vi "C867_Stop.vi"(8 "error in":errorcluster caption="entrée d'erreur") -> (0 "error out":errorcluster caption="sortie d'erreur")   [LabVIEW 2026]
uses:
  Controls/TypeDef_FGV.ctl
  C867-VIs/Low Level/PI_GCS2_DLL_x64.dll
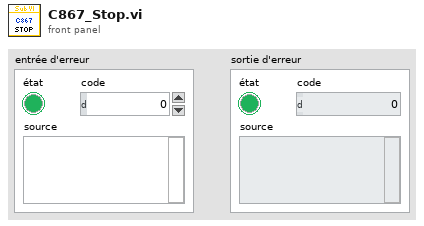
[diagram p1: front panel]
types:
  T1 = typedef "TypeDef_FGV.ctl" = enum16{"Initialize", "Write", "Read"}
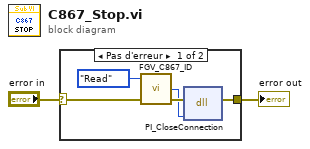
[diagram p0: block diagram]
diagram:
  n1 = case shown="Pas d'erreur" "error in" {
    selector: "error in" -> [w5 w8]
    tunnel: [w7 w8] -> w1
    frame No Error {
      n2 = call "FGV_C867_ID.vi"("error in"=w5, "Action"=TypeDef_FGV."Read") -> ("error out"=w6:errorcluster, "ID"=w4:i32)  [unwired: 2 in]
      n3 = dll-call lib="D:/SEBASTIEN/GitHub/LABVIEW-Useful-codes/Device_control/PC-C867-IO Control/v0.1/SubVI/PI-C867/C867-VIs/Low Level/PI_GCS2_DLL_x64.dll" fn="PI_CloseConnection"(error in=w6, "ID"=w4) -> (error out=w7:errorcluster)  [unwired: 4 in, 1 out]
    }
    frame Error {
    }
  }
  "error out" <- w1
